vi "saveNumberedImage.vi"(6 "currentPos":dbl, 8 "error in (no error)":errorcluster, 9 "Image":T1, 10 "imageNumber":u32, 11 "folder":path) -> (0 "error out":errorcluster)   [LabVIEW 2014]
uses:
  <vilib>/vision/Image Controls.llb/IMAQ Image.ctl
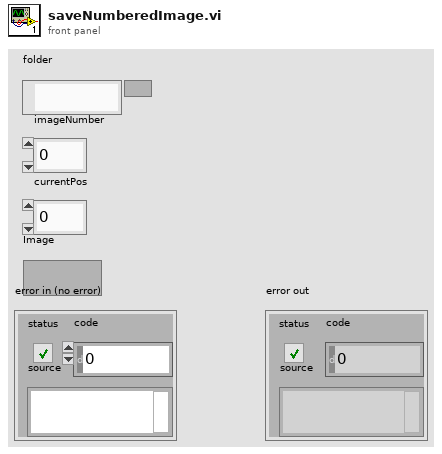
[diagram p1: front panel]
types:
  T1 = typedef "IMAQ Image.ctl" = refnum<image>
  T2 = enum16{"open", "replace", "create", "open or create", "replace or create", "replace or create with confirmation"}
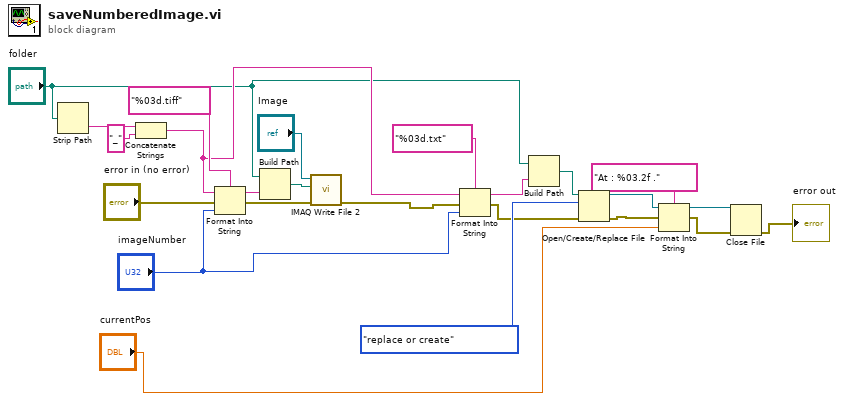
[diagram p0: block diagram]
diagram:
  n1 = Strip Path(path="folder") -> (name=w19:string)  [unwired: 1 out]
  n2 = Concatenate Strings(w19, "_" ("string")) -> (w12:string)
  n3 = Format Into String(format string="%03d.tiff", initial string=w12, error in="error in (no error)", "imageNumber") -> (resulting string=w23:string, error out=w21:errorcluster)
  n4 = Build Path(base path="folder", name or relative path=w23) -> (appended path=w22:path)
  n5 = call-poly "IMAQ Write File 2"("error in (no error)"=w21, "File Path"=w22, "Image"="Image") -> ("error out"=w15:errorcluster)  [unwired: 7 in, 1 out]
  n6 = Format Into String(format string="%03d.txt", initial string=w12, error in=w15, "imageNumber") -> (resulting string=w11:string, error out=w14:errorcluster)
  n7 = Build Path(base path="folder", name or relative path=w11) -> (appended path=w9:path)
  n8 = Open/Create/Replace File(file path (use dialog)=w9, error in=w14, operation (0:open)=T2."replace or create") -> (refnum out=w7:refnum<file>, error out=w8:errorcluster)  [unwired: 3 in, 1 out]
  n9 = Format Into String(format string="At : %03.2f .", initial string=w7, error in=w8, "currentPos") -> (resulting string=w3:refnum<file>, error out=w5:errorcluster)
  n10 = Close File(refnum=w3, error in=w5) -> (error out=→"error out":errorcluster)  [unwired: 1 out]
